vi "Account Database.vi"(7 "Command":T2, 8 "error in (no error)":errorcluster, 11 "Balance or Account #":u32) -> (0 "error out":errorcluster, 2 "Owned Record?":bool, 3 "Record":T1)   [LabVIEW 2011]
uses:
  TypeDefs/Simulated Database Command.ctl
  TypeDefs/Record.ctl
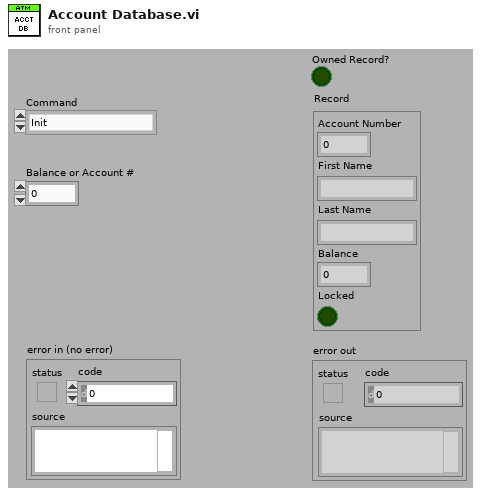
[diagram p1: front panel]
types:
  T1 = typedef "Record.ctl" = cluster{"Account Number":u32, "First Name":string, "Last Name":string, "Balance":dbl, "Locked":bool}
  T2 = typedef "Simulated Database Command.ctl" = enum16{"Init", "Look up and Lock Account", "Modify Balance", "Get Record", "Commit Record", "Unlock Record", "Close"}
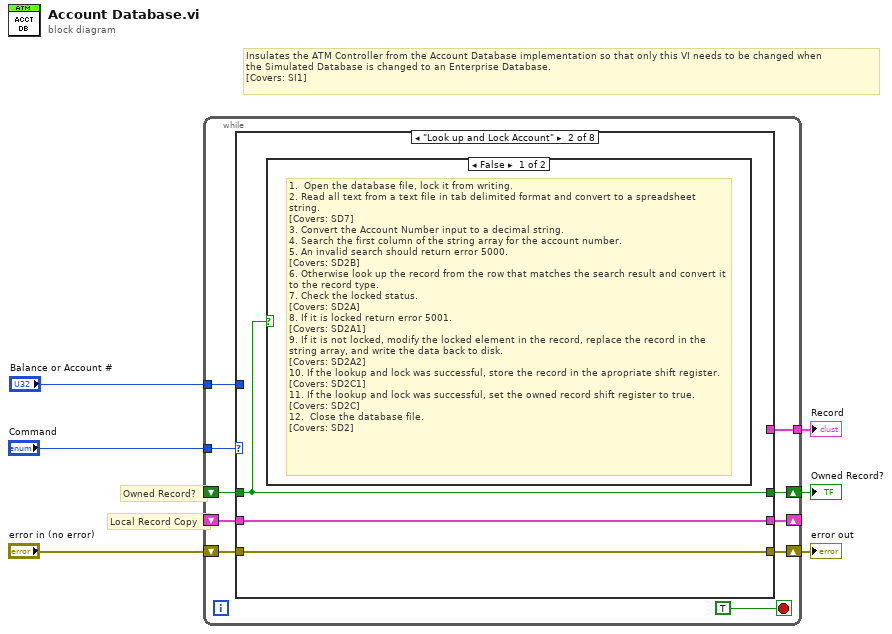
[diagram p0: block diagram]
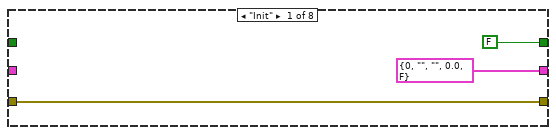
[diagram p2: hidden frame]
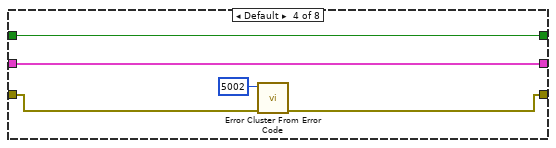
[diagram p6: hidden frame]
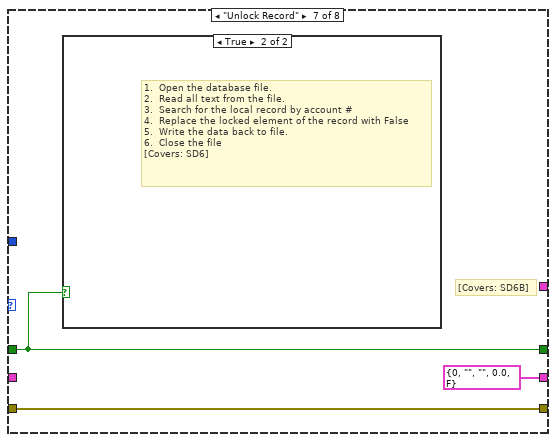
[diagram p11: hidden frame]
diagram:
  # "Insulates the ATM Controller from the Account Database implementation so that only this VI needs to be changed when\nthe Simulated Database is changed to an Enterprise Database.\n[Covers: SI1]"
  # "Local Record Copy"
  # "Owned Record?"
  n1 = while {
    tunnel: "Command" -> [w15]
    shift-right: [w13] -> w4
    shift-left: "error in (no error)" -> [w14]
    shift-right: [w12] -> _
    shift-left: _ -> [w11]
    shift-right: [w10] -> w2
    shift-left: _ -> [w9]
    tunnel: [w8] -> w3
    tunnel: "Balance or Account #" -> [w7]
    stop <- TRUE stop-if-true
    n2 = case shown="\"Look up and Lock Account\"" w15 {
      tunnel: w14 -> [w17 w22 w27 w32 w38 w43 w47 w50]
      tunnel: [w17 w22 w27 w31 w38 w43 w47 w50] -> w13
      tunnel: [T1 {"Account Number"=0, "First Name"="", "Last Name"="", "Balance"=0.0, "Locked"=FALSE} ("Record") w21 w24 w34 w37 w41 T1 {"Account Number"=0, "First Name"="", "Last Name"="", "Balance"=0.0, "Locked"=FALSE} ("Record") w49] -> w12
      tunnel: w11 -> [_ w21 w25 w34 w37 w41 _ w49]
      tunnel: [FALSE w20 w26 w33 w35 w42 w46 w48] -> w10
      tunnel: w9 -> [_ w20 w26 w33 w35 w42 w46 w48]
      tunnel: [_ _ w23 _ w36 w40 _ _] -> w8
      tunnel: w7 -> [_ _ _ _ _ _ _ _]
      frame "Init" {
      }
      frame "Look up and Lock Account" {
        n3 = case shown="False" w20 {
          frame False {
            # "1.  Open the database file, lock it from writing.\n2. Read all text from a text file in tab delimited format and convert to a spreadsheet string.\n[Covers: SD7]\n3. Convert the Account Number input to a decimal string.\n4. Search the first column of the string array for the account number.\n5. An invalid search should return error 5000.\n[Covers: SD2B]\n6. Otherwise look up the record from the row that matches the search result and convert it to the record type.\n7. Check the locked status.\n[Covers: SD2A]\n8. If it is locked return error 5001.\n[Covers: SD2A1]\n9. If it is not locked, modify the locked element in the record, replace the record in the string array, and write the data back to disk.\n[Covers: SD2A2]\n10. If the lookup and lock was successful, store the record in the apropriate shift register.\n[Covers: SD2C1]\n11. If the lookup and lock was successful, set the owned record shift register to true.\n[Covers: SD2C]\n12.  Close the database file.\n[Covers: SD2]"
          }
          frame True {
            # "Throw a session error.\n[Covers: SD2C2A]\n[Covers: SD2C2]"
          }
        }
      }
      frame "Modify Balance" {
        n4 = case shown="False" w26 {
          tunnel: [w28 w29] -> w24
          tunnel: w25 -> [w28 w29]
          tunnel: [_ w29] -> w23
          frame False {
            # "Throw a transaction error.\n[Covers: SD3A]"
          }
          frame True {
            # "Replace the balance element of the local record with the incoming balance.\n[Covers: SD3B]\n[Covers: SD3]"
          }
        }
      }
      frame Default {
        n5 = call <vilib>:"Error Cluster From Error Code.vi"("error in (no error)"=w32, "error code (0)"=5002) -> ("error out"=w31:errorcluster)  [unwired: 7 in]
      }
      frame "Get Record" {
        n6 = case shown="True" w35 {
          tunnel: [_ w39] -> w36
          tunnel: w37 -> [_ w39]
          frame False {
            # "Throw a transaction error.\n[Covers: SD4A]"
          }
          frame True {
            # "[Covers: SD4]"
          }
        }
      }
      frame "Commit Record" {
        n7 = case shown="True" w42 {
          tunnel: w41 -> [_ w44]
          tunnel: [_ w44] -> w40
          frame False {
            # "Throw a transaction error.\n[Covers: SD5A]"
          }
          frame True {
            # "1.  Open the database file.\n2.  Read all text from the file.\n3.  Search for the local record by account #\n4.  Replace the record in the string array\n5.  Write the data back to file.\n6.  Close the file\n[Covers: SD5B]  \n[Covers: SD5]"
          }
        }
      }
      frame "Unlock Record" {
        # "[Covers: SD6B]"
        n8 = case shown="True" w46 {
          frame False {
            # "Thow a session error.\n[Covers: SD6A]"
          }
          frame True {
            # "1.  Open the database file.\n2.  Read all text from the file.\n3.  Search for the local record by account #\n4.  Replace the locked element of the record with False\n5.  Write the data back to file.\n6.  Close the file\n[Covers: SD6]"
          }
        }
      }
      frame "Close" {
        # "Close the file reference"
      }
    }
  }
  "Record" <- w3
  "error out" <- w4
  "Owned Record?" <- w2
